vi "test CAN Cyclic Outgoing with Disable and Trigger Channels.vi"(8 "error in (no error)":errorcluster, 11 "TestCase in":refnum<class "CAN Outgoing Tests.lvclass">) -> (0 "error out":errorcluster, 3 "TestCase out":refnum<class "CAN Outgoing Tests.lvclass">)   [LabVIEW 2017, in "CAN Outgoing Tests.lvclass"]
uses:
  CAN Outgoing Tests.lvclass
  C:/Users/nitest/Documents/ni-official/niveristand-custom-device-testing-tools/VeriStandTestCase/VeriStandTestCase.lvclass
  CAN Outgoing Tests.lvclass/CAN Outgoing Tests.ctl
  25aeefa7-2a66-4394-b60b-98a5bb793f09.vi
  e87c5cb7-3d82-47e5-a716-e740ec705cc5.vi
  <vilib>/NI Veristand/Execution/Workspace/NI VeriStand - Set Multiple Channel Values.vi
  <vilib>/xnet/xnet.llb/XNET Read (Frame CAN).vi
  <vilib>/addons/_JKI Toolkits/VI Tester/TestCase.llb/TestCase.lvclass
  <vilib>/NI VeriStand/Execution/Workspace/NI_VS Workspace ExecutionAPI.lvlib
  C:/Program Files (x86)/National Instruments/LabVIEW 2017/vi.lib/addons/_JKI Toolkits/VI Tester/TestCase.llb/TestCase.lvclass
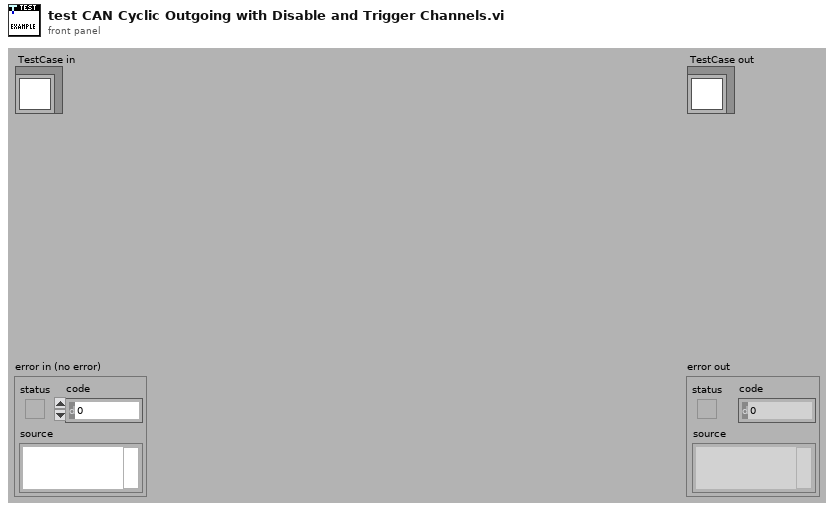
[diagram p1: front panel]
types:
  T1 = cluster{"Disable Frame?":bool, "Enable Oscillator?":bool, "Oscillator Frequency":dbl, "Expected Number of Frames":i32}[]
  T2 = typedef "NI_VS Workspace ExecutionAPI.lvlib/WorkspaceAPI.ctl" = refnum<k24>
  T3 = typedef "XNET Frame CAN.ctl" = cluster{"timestamp":timestamp, "payload":u8[], "identifier":u32, "type":T4, "extended?":bool, "echo?":bool}
  T4 = typedef "XNET Frame Type CAN.ctl" = u8
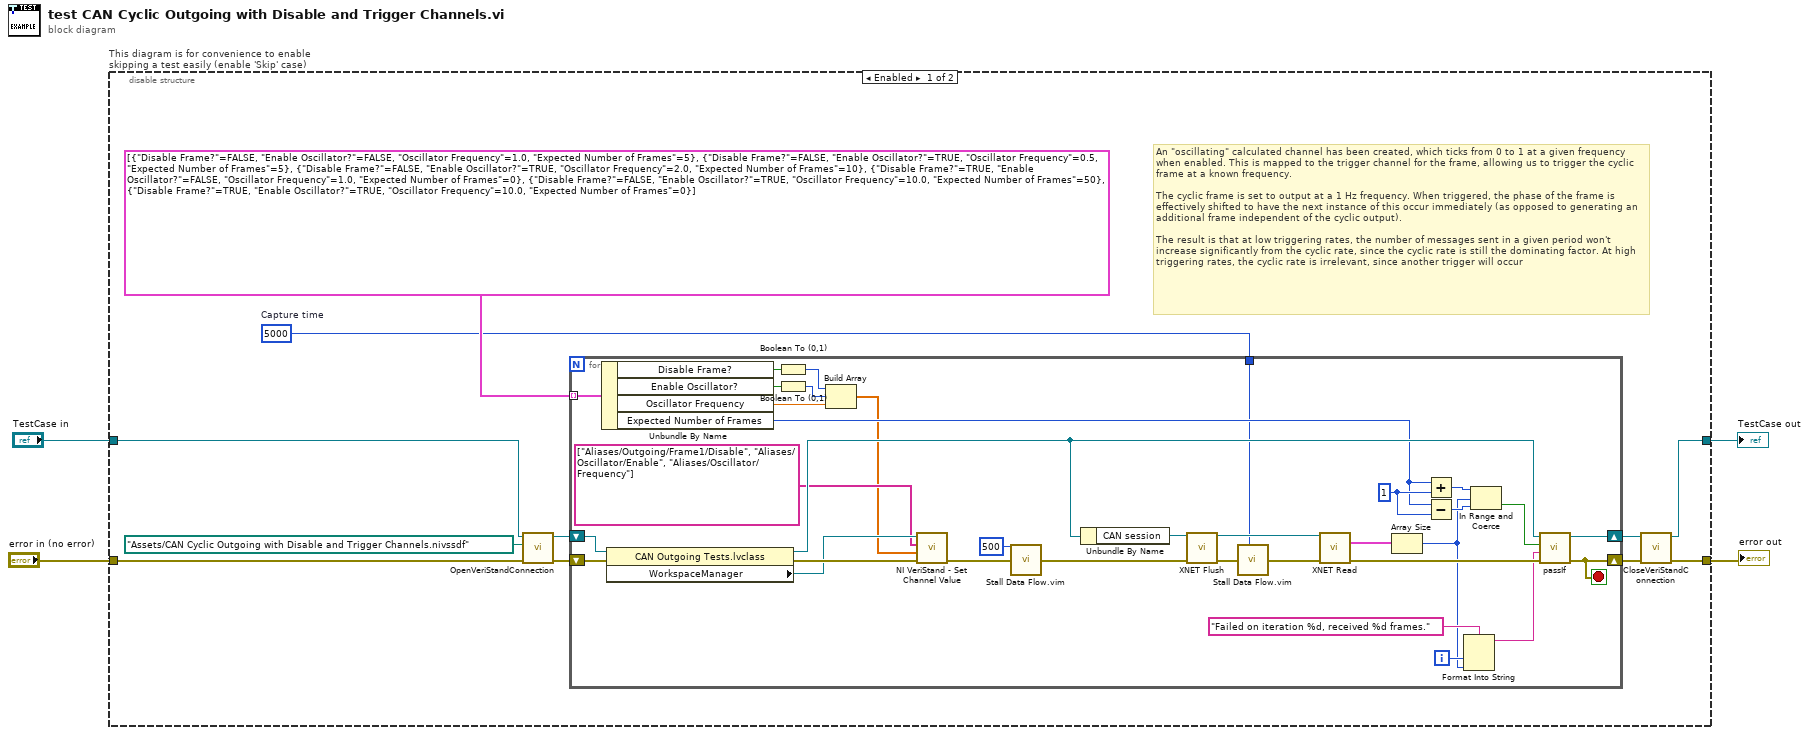
[diagram p0: block diagram]
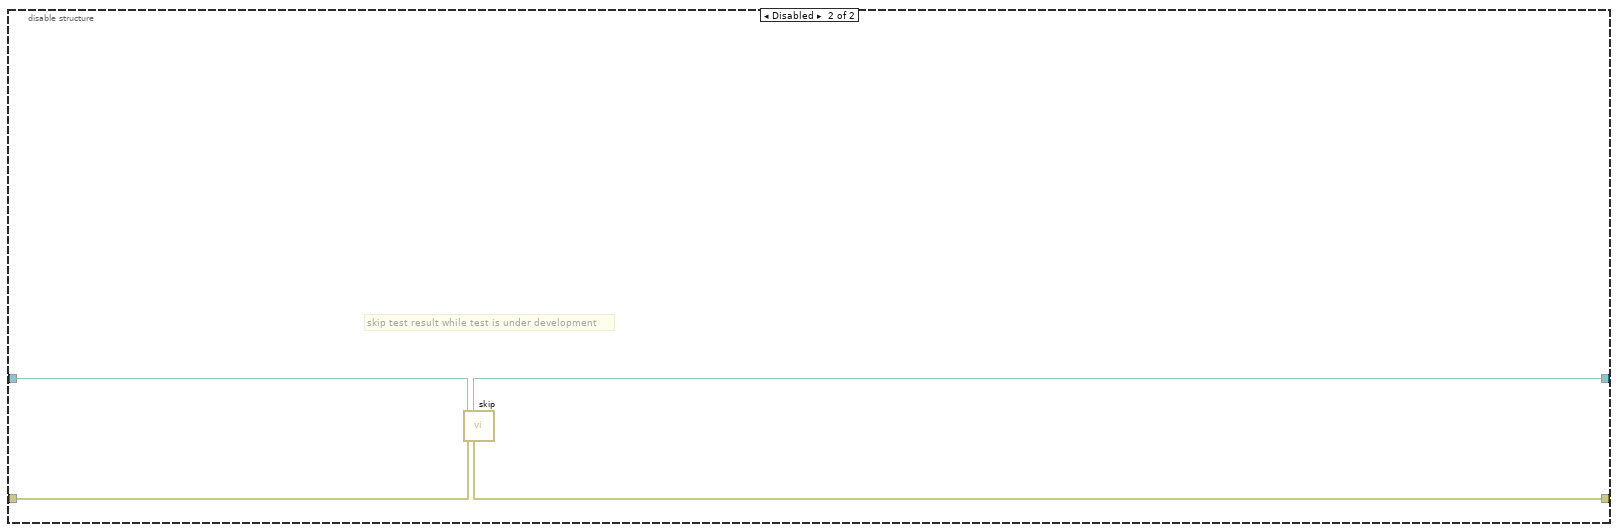
[diagram p2: hidden frame]
diagram:
  n1 = disable-structure "This diagram is for convenience to enable skipping a test easily (enable 'Skip' case)" shown="Enabled" {
    disable-tunnel: "TestCase in" -> [w12 w53]
    disable-tunnel: [w7 w51] -> w1
    disable-tunnel: [w9 w52] -> w3
    disable-tunnel: "error in (no error)" -> [w14 w50]
    frame Enabled {
      w5 = u32 5000  # Capture time
      # "An \"oscillating\" calculated channel has been created, which ticks from 0 to 1 at a given frequency when enabled. This is mapped to the trigger channel for the frame, allowing us to trigger the cyclic frame at a known frequency.\n\nThe cyclic frame is set to output at a 1 Hz frequency. When triggered, the phase of the frame is effectively shifted to have the next instance of this occur immediately (as opposed to generating an additional frame independent of the cyclic output).\n\nThe result is that at low triggering rates, the number of messages sent in a given period won't increase significantly from the cyclic rate, since the cyclic rate is still the dominating factor. At high triggering rates, the cyclic rate is irrelevant, since another trigger will occur"
      n2 = call-dynamic "OpenVeriStandConnection.vi"("error in (no error)"=w14, "System Definition File"=path "Assets/CAN Cyclic Outgoing with Disable and Trigger Channels.nivssdf", "VeriStand Test Case in"=w12) -> ("error out"=w13:errorcluster, "VeriStand Test Case out"=w11:refnum<class "CAN Outgoing Tests.lvclass">)  [unwired: 6 in, 1 out]
      n3 = for {
        shift-right: [w25] -> w15
        shift-left: w13 -> [w39]
        shift-right: [w40] -> w8
        shift-left: w11 -> [w37]
        tunnel: T1 [{"Disable Frame?"=FALSE, "Enable Oscillator?"=FALSE, "Oscillator Frequency"=1.0, "Expected Number of Frames"=5}, {"Disable Frame?"=FALSE, "Enable Oscillator?"=TRUE, "Oscillator Frequency"=0.5, "Expected Number of Frames"=5}, {"Disable Frame?"=FALSE, "Enable Oscillator?"=TRUE, "Oscillator Frequency"=2.0, "Expected Number of Frames"=10}, {"Disable Frame?"=TRUE, "Enable Oscillator?"=FALSE, "Oscillator Frequency"=1.0, "Expected Number of Frames"=0}, {"Disable Frame?"=FALSE, "Enable Oscillator?"=TRUE, "Oscillator Frequency"=10.0, "Expected Number of Frames"=50}, {"Disable Frame?"=TRUE, "Enable Oscillator?"=TRUE, "Oscillator Frequency"=10.0, "Expected Number of Frames"=0}] -> [w23] mode=indexing
        tunnel: w5 -> [w24]
        i -> [w20]
        stop <- w25 stop-if-true
        w42 = 1
        n4 = Unbundle By Name(w23) -> ("Disable Frame?"=w17:bool, "Enable Oscillator?"=w31:bool, "Oscillator Frequency"=w29:dbl, "Expected Number of Frames"=w33:i32)
        n5 = property class="CAN Outgoing Tests.lvclass"(reference=w37, error in=w39) -> (reference out=w36:refnum<class "CAN Outgoing Tests.lvclass">, error out=w38:errorcluster, "WorkspaceManager"=w34:T2)
        n6 = Boolean To (0,1)(Boolean=w17) -> (0, 1=w16:i16)
        n7 = Boolean To (0,1)(Boolean=w31) -> (0, 1=w30:i16)
        n8 = Build Array(w16, w30, w29) -> (w28:dbl[])
        n9 = call-poly <vilib>:"NI VeriStand - Set Channel Value.vi"("error in (no error)"=w38, "Values"=w28, "Channels"=string[] ["Aliases/Outgoing/Frame1/Disable", "Aliases/Oscillator/Enable", "Aliases/Oscillator/Frequency"], "WorkspaceManager in"=w34) -> ("error out"=w35:errorcluster)  [unwired: 6 in, 1 out]
        n10 = call "Stall Data Flow.vim"("value in"=w35, "milliseconds to wait"=u32 500) -> ("value out"=w27:errorcluster)  [unwired: 1 out]
        n11 = Unbundle By Name(w36) -> ("CAN session"=w49:refnum<k21>)
        n12 = call <vilib>:"XNET Flush.vi"("session in"=w49, "error in (no error)"=w27) -> ("session out"=w46:refnum<k21>, "error out"=w47:errorcluster)  [unwired: 12 in]
        n13 = call "Stall Data Flow.vim"("value in"=w47, "milliseconds to wait"=w24) -> ("value out"=w48:errorcluster)  [unwired: 1 out]
        n14 = call-poly <vilib>:"XNET Read.vi"("session in"=w46, "error in (no error)"=w48) -> ("data"=w22:T3[], "error out"=w45:errorcluster)  [unwired: 10 in, 2 out]
        n15 = Array Size(array=w22) -> (size(s)=w19:i32)
        n16 = Add(x=w33, y=w42) -> (x+y=w44:i32)
        n17 = Subtract(x=w33, y=w42) -> (x-y=w43:i32)
        n18 = Format Into String(format string="Failed on iteration %d, received %d frames.", w20, w19) -> (resulting string=w18:string)  [unwired: 2 in, 1 out]
        n19 = In Range and Coerce(upper limit=w44, x=w19, lower limit=w43) -> (In Range?=w41:bool)  [unwired: 1 out]
        n20 = call-dynamic "passIf.vi"("error in (no error)"=w45, "message (\"\")"=w18, "pass"=w41, "TestCase in"=w36) -> ("error out"=w25:errorcluster, "TestCase out"=w40:refnum<class "CAN Outgoing Tests.lvclass">)  [unwired: 6 in]
      }
      n21 = call-dynamic "CloseVeriStandConnection.vi"("error in (no error)"=w15, "VeriStand Test Case in"=w8) -> ("error out"=w9:errorcluster, "VeriStand Test Case out"=w7:refnum<class "CAN Outgoing Tests.lvclass">)  [unwired: 8 in]
    }
    frame Disabled {
      # "skip test result while test is under development"
      n22 = call <vilib>:"skip.vi"("error in (no error)"=w50, "TestCase in"=w53) -> ("error out"=w52:errorcluster, "TestCase out"=w51:refnum<class "CAN Outgoing Tests.lvclass">)  [unwired: 8 in]
    }
  }
  "error out" <- w3
  "TestCase out" <- w1
